vi "cov_corr(SubVI).vi"(10 "Gaussian noise pattern 2":dbl[](array[numeric]), 11 "Gaussian noise pattern":dbl[](array[numeric])) -> (2 "korelacja":dbl, 3 "kowariancja":dbl)   [LabVIEW 2025]
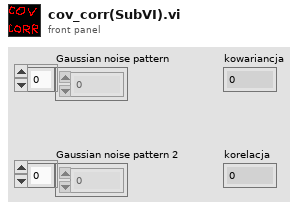
[diagram p1: front panel]
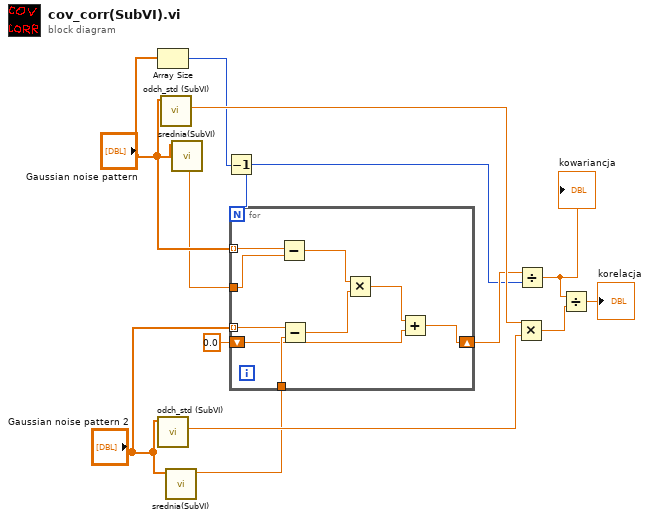
[diagram p0: block diagram]
diagram:
  n1 = Array Size(array="Gaussian noise pattern") -> (size(s)=w6:i32)
  n2 = call "odch_std (SubVI).vi"("Gaussian noise pattern"="Gaussian noise pattern 2") -> ("odchylenie standardowe"=w8:dbl)  [unwired: 9 in, 1 out]
  n3 = call "odch_std (SubVI).vi"("Gaussian noise pattern"="Gaussian noise pattern") -> ("odchylenie standardowe"=w9:dbl)  [unwired: 9 in, 1 out]
  n4 = call "srednia(SubVI).vi"("input"="Gaussian noise pattern 2") -> ("arytm"=w3:dbl)  [unwired: 8 in, 2 out]
  n5 = call "srednia(SubVI).vi"("input"="Gaussian noise pattern") -> ("arytm"=w4:dbl)  [unwired: 8 in, 2 out]
  n6 = Decrement(x=w6) -> (x-1=w1:i32)
  n7 = for {
    N: w1 -> [_]
    tunnel: "Gaussian noise pattern" -> [w22] mode=indexing
    tunnel: "Gaussian noise pattern 2" -> [w21] mode=indexing
    tunnel: w3 -> [w20]
    tunnel: w4 -> [w19]
    shift-right: [w14] -> w5
    shift-left: 0.0 -> [w16]
    n8 = Subtract(x=w22, y=w19) -> (x-y=w18:dbl)
    n9 = Subtract(x=w21, y=w20) -> (x-y=w17:dbl)
    n10 = Multiply(x=w18, y=w17) -> (x*y=w15:dbl)
    n11 = Add(x=w15, y=w16) -> (x+y=w14:dbl)
  }
  n12 = Multiply(x=w9, y=w8) -> (x*y=w11:dbl)
  n13 = Divide(x=w5, y=w1) -> (x/y=w10:dbl)
  "kowariancja" <- w10
  n14 = Divide(x=w10, y=w11) -> (x/y=→"korelacja":dbl)
